vi "End Live Stream.vi"(8 "error in":errorcluster, 11 "IMG_SRC in":refnum<class "IMG_SRC.lvclass">) -> (0 "error out":errorcluster, 3 "IMG_SRC out":refnum<class "IMG_SRC.lvclass">)   [LabVIEW 2018, in "IMG_SRC.lvlib" / "IMG_SRC.lvclass"]
uses:
  IMG_SRC.lvclass
  IMG_SRC.lvclass/IMG_SRC.ctl
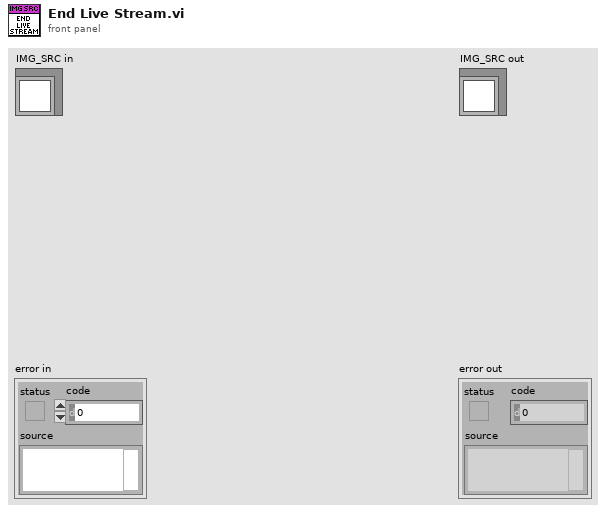
[diagram p1: front panel]
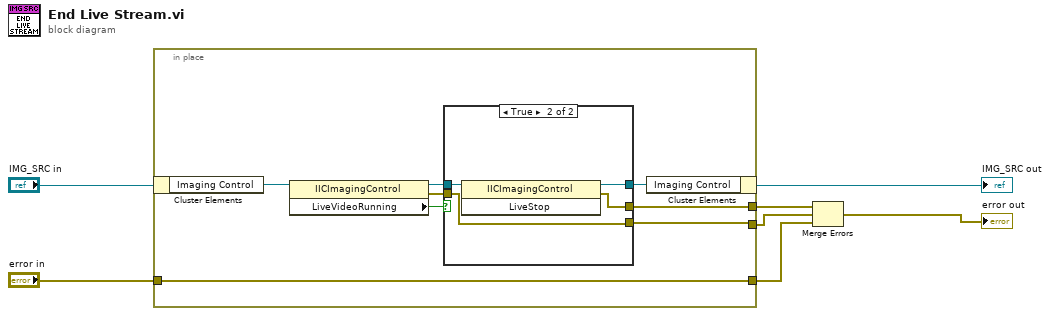
[diagram p0: block diagram]
diagram:
  n1 = in-place {
    in-place-border: [w9] -> w5
    in-place-border: "error in" -> [w10]
    in-place-border: [w10] -> w1
    in-place-border: [w8] -> w2
    n2 = in-place-cluster #1("IMG_SRC in") -> ("Imaging Control"=w12:refnum<k7>)
    n3 = property class="IICImagingControl"(reference=w12) -> (reference out=w14:refnum<k7>, error out=w13:errorcluster, "LiveVideoRunning"=w15:bool)  [unwired: 1 in]
    n4 = case shown="True" w15 {
      tunnel: w14 -> [w17 w21]
      tunnel: w13 -> [w16 w19]
      tunnel: [w17 w20] -> w11
      tunnel: [w16 w19] -> w8
      tunnel: [w16 w18] -> w9
      frame False {
      }
      frame True {
        n5 = invoke class="IICImagingControl" method="LiveStop"(reference=w21) -> (reference out=w20:refnum<k7>, error out=w18:errorcluster)  [unwired: 2 in, 1 out]
      }
    }
    n6 = in-place-cluster #1("Imaging Control"=w11) -> (→"IMG_SRC out":refnum<class "IMG_SRC.lvclass">)
  }
  n7 = Merge Errors(w5, w2, w1) -> (→"error out":errorcluster)
